vi "Configure Motor Electrical Angle.vi"(6 "Manual Correction Value (0.00)":i32 min=-180 max=180 format="%.2f", 7 "Enable Electrical Angle Measurement (T: Enable)":bool=TRUE, 8 "error in (no error)":errorcluster, 9 "Auto Enter Target (0: U1)":i32(ring) items=["U1", "I1", "U2", "I2", "U3", "I3", "U4", "I4", "U5", "I5", "U6", "I6"], 10 "Enable Auto Enter Correction (T: Enable)":bool=TRUE, 11 "VISA resource name":refnum<visa-resource-name>) -> (0 "error out":errorcluster, 3 "VISA resource name out":refnum<visa-resource-name>)   [LabVIEW 2021, in "Yokogawa WT1800 Series.lvlib"]
doc: "Configures the motor electrical angle features.\n\n<b>Note:</b>\nThis setting valid on models with the motor evaluation function (/MTR) option,\nand the harmonic measurement (/G5 or /G6) option."
uses:
  <instrlib>/Yokogawa WT1800 Series/Yokogawa WT1800 Series.lvlib
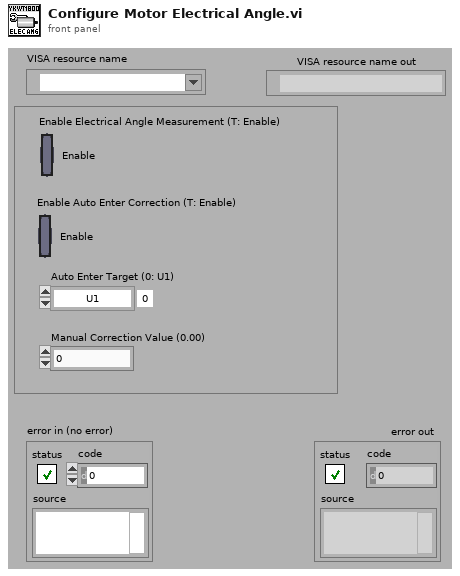
[diagram p1: front panel]
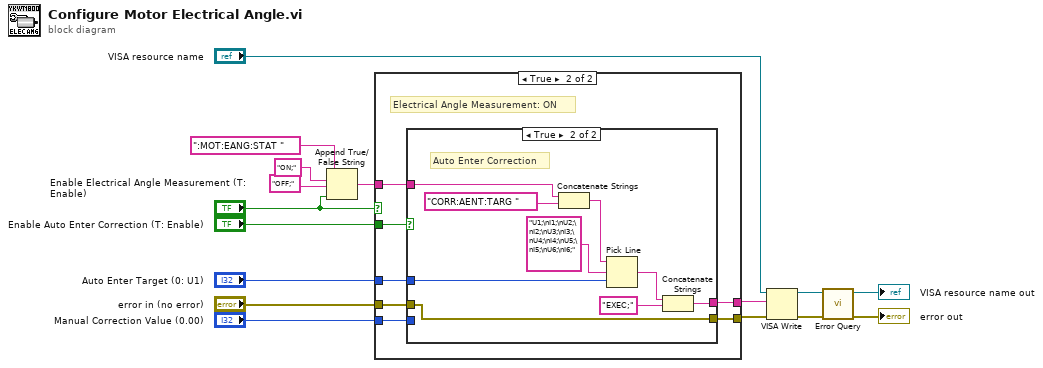
[diagram p0: block diagram]
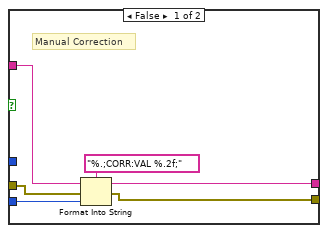
[diagram p3: hidden frame]
diagram:
  n1 = Append True/False String ("True/False 文字列を追加")(1:"Enable Electrical Angle Measurement (T: Enable)", 2:"OFF;", 3:"ON;", 4:":MOT:EANG:STAT " ("¶ñi\"\"j")) -> (0:w5:string)
  n2 = case shown="True" "Enable Electrical Angle Measurement (T: Enable)" {
    tunnel: "Manual Correction Value (0.00)" -> [_ w25]
    tunnel: "error in (no error)" -> [w17 w24]
    tunnel: w5 -> [w18 w23]
    tunnel: [w18 w22] -> w4
    tunnel: [w17 w21] -> w3
    tunnel: "Enable Auto Enter Correction (T: Enable)" -> [_ w20]
    tunnel: "Auto Enter Target (0: U1)" -> [_ w19]
    frame False {
      # "Electrical Angle Measurement: OFF"
    }
    frame True {
      # "Electrical Angle Measurement: ON"
      n3 = case shown="True" w20 {
        tunnel: w25 -> [w30 _]
        tunnel: w24 -> [w29 w33]
        tunnel: w23 -> [w28 w39]
        tunnel: [w27 w34] -> w22
        tunnel: [w26 w33] -> w21
        tunnel: w19 -> [_ w32]
        frame False {
          # "Manual Correction"
          n4 = Format Into String(format string="%.;CORR:VAL %.2f;" ("形式文字列"), initial string=w28, error in=w29, w30) -> (resulting string=w27:string, error out=w26:errorcluster)
        }
        frame True {
          # "Auto Enter Correction"
          n5 = Concatenate Strings(w39, "CORR:AENT:TARG " ("文字列")) -> (w35:string)
          n6 = Pick Line ("ライン選択")(string ("")=w35, multi-line string="U1;\nI1;\nU2;\nI2;\nU3;\nI3;\nU4;\nI4;\nU5;\nI5;\nU6;\nI6;" ("複数行文字列"), line index=w32) -> (output string=w37:string)
          n7 = Concatenate Strings(w37, "EXEC;" ("出力文字列")) -> (w34:string)
        }
      }
    }
  }
  n8 = VISA Write ("VISA書き込み")(VISA resource name="VISA resource name", write buffer=w4, error in (no error)=w3) -> (VISA resource name out=w16:refnum<visa-resource-name>, error out=w15:errorcluster)  [unwired: 1 out]
  n9 = call <instrlib>:"Error Query.vi"("error in (no error)"=w15, "VISA resource name"=w16) -> ("error out"=→"error out":errorcluster, "VISA resource name out"=→"VISA resource name out":refnum<visa-resource-name>)  [unwired: 6 in, 2 out]
